vi "Save and close refs.vi"(8 "error in (no error)":errorcluster, 11 "SysDef Refs in":T1) -> (0 "error out":errorcluster)   [LabVIEW 2010]
uses:
  SysDefRefs.ctl
  NationalInstruments.VeriStand.SystemDefinitionAPI
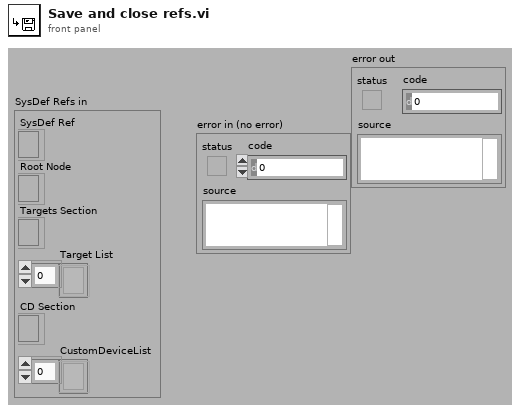
[diagram p1: front panel]
types:
  T1 = typedef "SysDefRefs.ctl" = cluster{"SysDef Ref":refnum<k24>, "Root Node":refnum<k24>, "Targets Section":refnum<k24>, "Target List":refnum<k24>[], "CD Section":refnum<k24>, "CustomDeviceList":refnum<k24>[]}
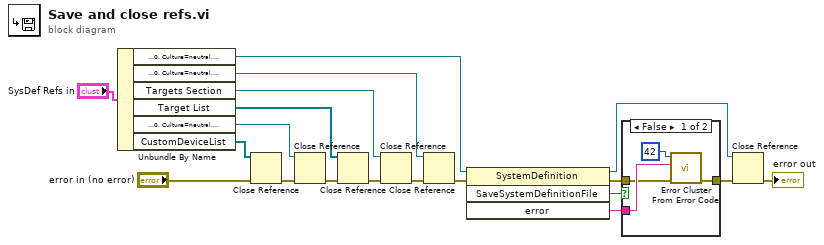
[diagram p0: block diagram]
diagram:
  n1 = Unbundle By Name("SysDef Refs in") -> ("SysDef Ref"=w5:refnum<k24>, "Root Node"=w6:refnum<k24>, "Targets Section"=w7:refnum<k24>, "Target List"=w8:refnum<k24>[], "CD Section"=w4:refnum<k24>, "CustomDeviceList"=w1:refnum<k24>[])
  n2 = Close Reference(reference=w1, error in (no error)="error in (no error)") -> (error out=w3:errorcluster)
  n3 = Close Reference(reference=w4, error in (no error)=w3) -> (error out=w16:errorcluster)
  n4 = Close Reference(reference=w8, error in (no error)=w16) -> (error out=w17:errorcluster)
  n5 = Close Reference(reference=w7, error in (no error)=w17) -> (error out=w18:errorcluster)
  n6 = Close Reference(reference=w6, error in (no error)=w18) -> (error out=w19:errorcluster)
  n7 = invoke class="SystemDefinition" method="SaveSystemDefinitionFile"(reference=w5, error in=w19) -> (reference out=w15:refnum<k24>, error out=w13:errorcluster, "SaveSystemDefinitionFile"=w11:bool, "error"=w12:string)  [unwired: 2 in]
  n8 = case shown="False" w11 {
    tunnel: w12 -> [w23 _]
    tunnel: [w21 w24] -> w14
    tunnel: w13 -> [w20 w24]
    frame False {
      n9 = call <vilib>:"Error Cluster From Error Code.vi"("error in (no error)"=w20, "error message (\"\")"=w23, "error code (0)"=42) -> ("error out"=w21:errorcluster)  [unwired: 6 in]
    }
    frame True {
    }
  }
  n10 = Close Reference(reference=w15, error in (no error)=w14) -> (error out=→"error out":errorcluster)
